vi "Repeat Buy BG - Read.vi"(8 "error in (no error)":errorcluster, 11 "Globals in":refnum<class "TSM Context Data Access.lvclass">) -> (0 "error out":errorcluster, 2 "Repeat Buy BG":bool[](array[boolean]), 3 "Globals out":refnum<class "TSM Context Data Access.lvclass">)   [LabVIEW 2019, in "TSM Context Data Access.lvclass"]
uses:
  TSM Context Data Access.lvclass
  TSM Context Data Access.lvclass/TSM Context Data Access.ctl
  <vilib>/NI_TestStand_SemiconductorModule/NI_TestStand_Semiconductor_Module.lvlibp
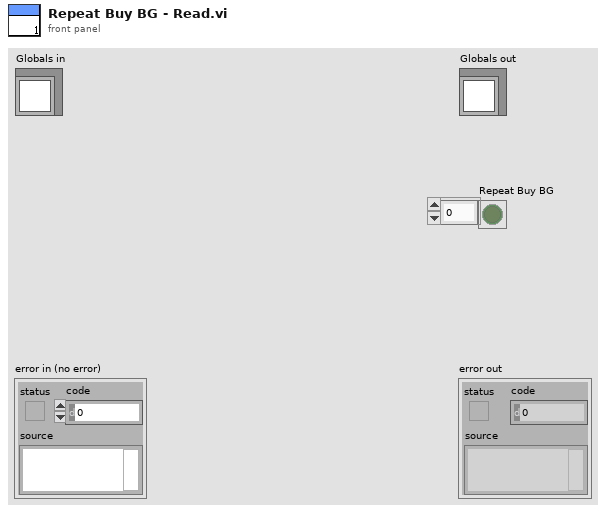
[diagram p1: front panel]
types:
  T1 = typedef "NI_TestStand_Semiconductor_Module.lvlibp/SemiconductorModuleContext.ctl" = refnum<k7>
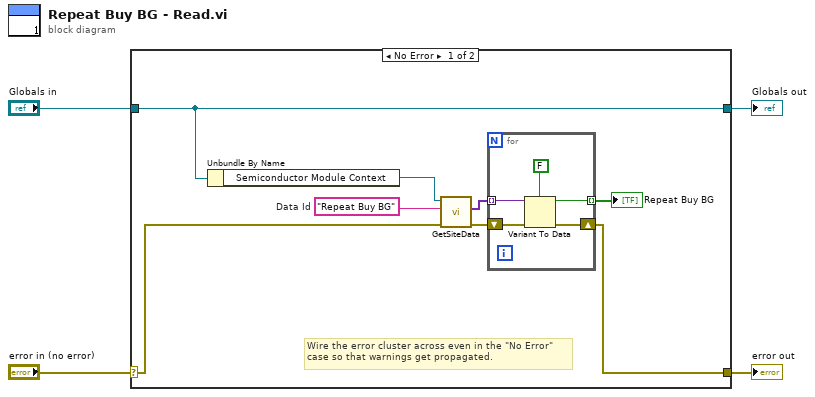
[diagram p0: block diagram]
diagram:
  n1 = case shown="No Error" "error in (no error)" {
    selector: "error in (no error)" -> [w7 w19]
    tunnel: [w6 w19] -> w3
    tunnel: [w8 w18] -> w1
    tunnel: "Globals in" -> [w8 w18]
    frame No Error {
      w10 = "Repeat Buy BG"  # Data Id
      # "Wire the error cluster across even in the \"No Error\"\ncase so that warnings get propagated."
      n2 = Unbundle By Name(w8) -> ("Semiconductor Module Context"=w11:T1)
      n3 = call <vilib>:"GetSiteData.vi"("error in (no error)"=w7, "Data Id"=w10, "Semiconductor Module Context"=w11) -> ("error out"=w12:errorcluster, "Site Data"=w9:variant[])  [unwired: 6 in, 1 out]
      n4 = for {
        tunnel: [w16] -> w5 mode=indexing
        tunnel: w9 -> [w14] mode=indexing
        shift-right: [w17] -> w6
        shift-left: w12 -> [w15]
        n5 = Variant To Data(error in=w15, type=FALSE, Variant=w14) -> (data=w16:bool, error out=w17:errorcluster)
      }
      "Repeat Buy BG" <- w5
    }
    frame Error {
    }
  }
  "error out" <- w3
  "Globals out" <- w1
